vi "getRef.vi"(8 "error in (no error)":errorcluster) -> (0 "error out":errorcluster, 2 "python_ref":refnum<class "python.lvclass">)   [LabVIEW 2014, in "python.lvclass"]
uses:
  python.lvclass
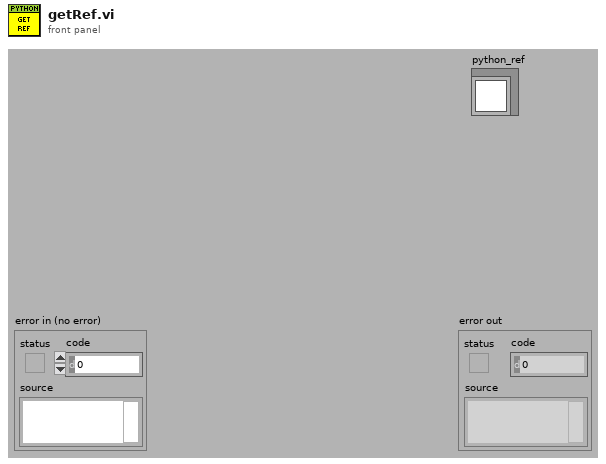
[diagram p1: front panel]
types:
  T1 = typedef "python.lvclass/ClassAttributesRef.ctl" = refnum<data-value>
  T2 = typedef "python.lvclass/ClassAttributes.ctl" = cluster{"Dummy":bool, "python_class":refnum<class "python.lvclass">[]}
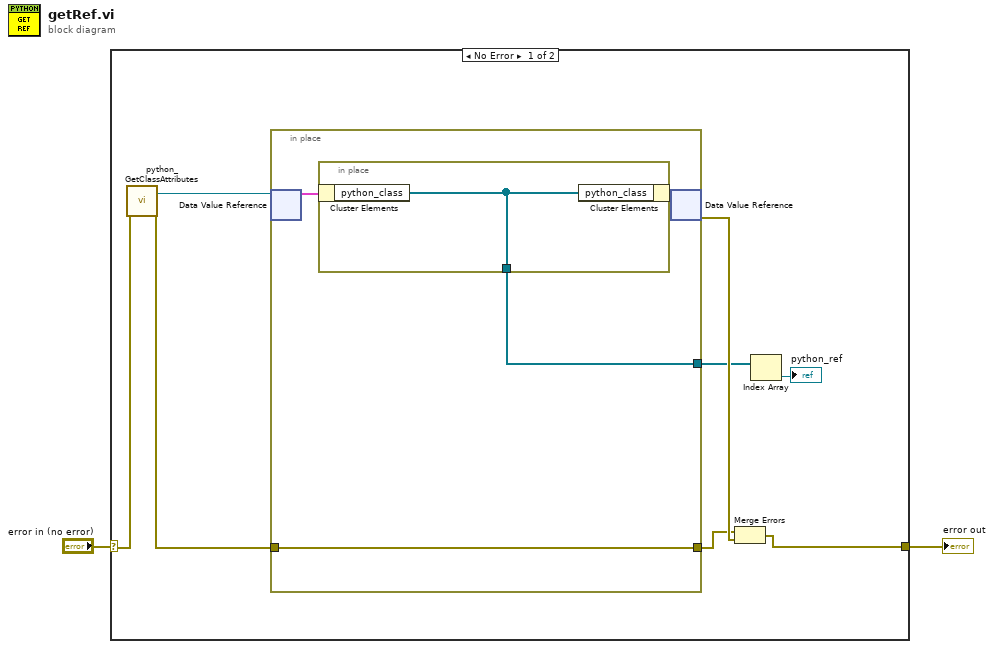
[diagram p0: block diagram]
diagram:
  n1 = case shown="No Error" "error in (no error)" {
    selector: "error in (no error)" -> [w7 w16]
    tunnel: [w10 w16] -> w1
    frame No Error {
      n2 = call "python_GetClassAttributes.vi"("error in (no error)"=w7) -> ("class attributes ref"=w5:T1, "error out"=w6:errorcluster)  [unwired: 15 in, 2 out]
      n3 = in-place {
        in-place-border: w6 -> [w12]
        in-place-border: [w12] -> w8
        in-place-border: [w11] -> w4
        n4 = in-place-dvr #1(w5) -> (w13:T2)  [unwired: 1 out]
        n5 = in-place {
          in-place-border: [w15] -> w11
          n6 = in-place-cluster #2(w13) -> ("python_class"=w15:refnum<class "python.lvclass">[])
          n7 = in-place-cluster #2("python_class"=w15) -> (w14:T2)
        }
        n8 = in-place-dvr #1(w14) -> (w9:errorcluster)  [unwired: 1 out]
      }
      n9 = Merge Errors(w8, w9) -> (w10:errorcluster)
      n10 = Index Array(array=w4) -> (element=→"python_ref":refnum<class "python.lvclass">)  [unwired: 1 in]
    }
    frame Error {
    }
  }
  "error out" <- w1
